vi "Test-Timevi.vi"() -> ()   [LabVIEW 2014]
panel:
  out "min":dbl
  out "结束时间":timestamp
  out "开始时间":timestamp
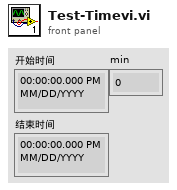
[diagram p1: front panel]
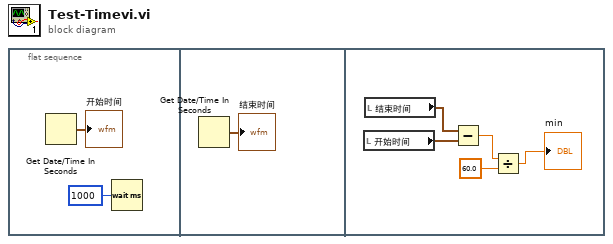
[diagram p0: block diagram]
diagram:
  n1 = flat-sequence {
    frame #0 {
      n2 = Get Date/Time In Seconds() -> (seconds since 1Jan1904=→"开始时间":timestamp)
      n3 = Wait (ms)(milliseconds to wait=u32 1000 ("等待时间（毫秒）")) -> ()  [unwired: 1 out]
    }
    frame #1 {
      n4 = Get Date/Time In Seconds() -> (seconds since 1Jan1904=→"结束时间":timestamp)
    }
    frame #2 {
      n5 = local read "开始时间"() -> (w7:timestamp)
      n6 = local read "结束时间"() -> (w8:timestamp)
      n7 = Subtract(x=w8, y=w7) -> (x-y=w5:dbl)
      n8 = Divide(x=w5, y=60.0) -> (x/y=→"min":dbl)
    }
  }
